vi "Get Software Set Config.vi"(8 "error in (no error)":errorcluster) -> (0 "error out":errorcluster, 2 "add on guids":string[](array[string]), 3 "software set guid":string)   [LabVIEW 2013]
uses:
  globals/Globals.vi
  <vilib>/Utility/config.llb/Read Key (String).vi
  <vilib>/Utility/sysdir.llb/Get System Directory.vi
  <vilib>/Utility/config.llb/NI_LVConfig.lvlib
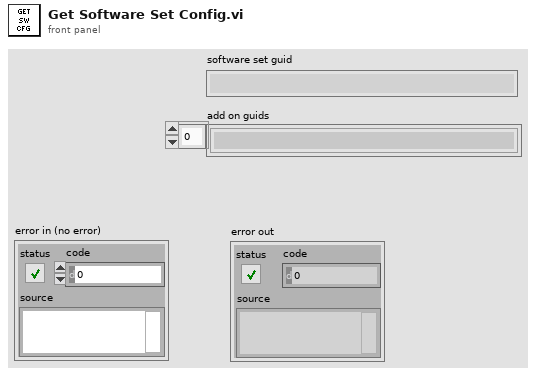
[diagram p1: front panel]
types:
  T1 = typedef "NI_LVConfig.lvlib/Config Data RefNum.ctl" = refnum<k1>
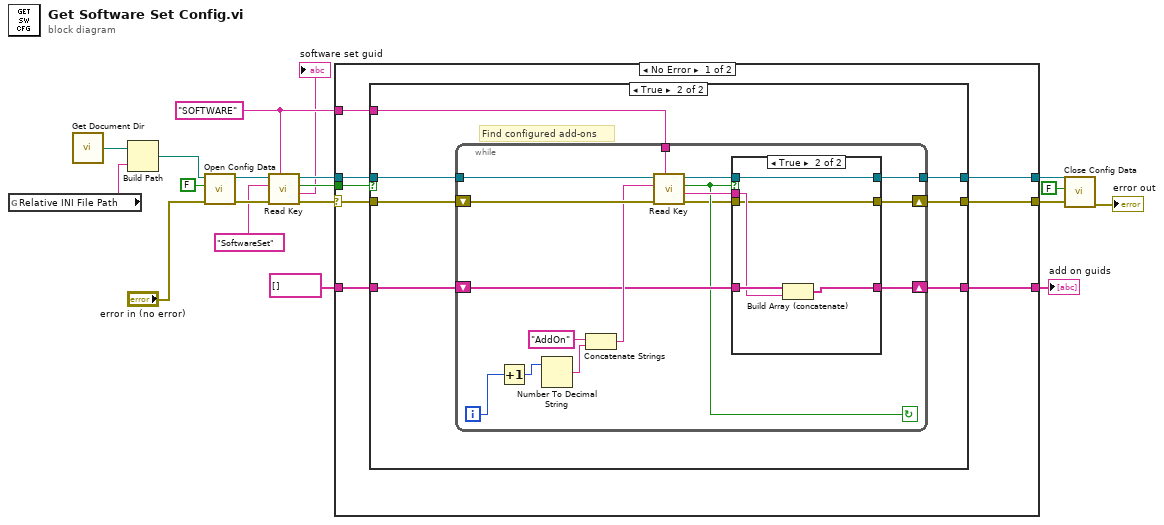
[diagram p0: block diagram]
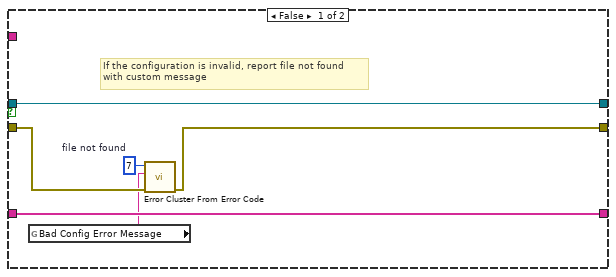
[diagram p2: hidden frame]
diagram:
  w19 = "SOFTWARE" ("section")
  n1 = global read "Globals.vi" "Relative INI File Path"() -> (w13:string)
  n2 = call "Get Document Dir.vi"() -> ("document dir"=w14:path)
  n3 = Build Path(base path=w14, name or relative path=w13) -> (appended path=w12:path)
  n4 = call <vilib>:"Open Config Data.vi"("error in (no error)"="error in (no error)", "create file if necessary (T)"=FALSE, "configuration file path"=w12) -> ("error out"=w16:errorcluster, "refnum"=w17:T1)  [unwired: 6 in, 1 out]
  n5 = call-poly <vilib>:"Read Key.vi"("section"=w19, "error in (no error)"=w16, "key"="SoftwareSet", "refnum"=w17) -> ("error out"=w9:errorcluster, "value"=→"software set guid":string, "found?"=w11:bool, "refnum out"=w10:T1)  [unwired: 4 in]
  n6 = case shown="No Error" w9 {
    selector: w9 -> [w25 w66]
    tunnel: w11 -> [w27 _]
    tunnel: w10 -> [w26 w67]
    tunnel: w19 -> [w24 _]
    tunnel: string[] [] -> [w23 w65]
    tunnel: [w22 w65] -> w5
    tunnel: [w21 w66] -> w4
    tunnel: [w20 w67] -> w3
    frame No Error {
      n7 = case shown="True" w27 {
        tunnel: w26 -> [w28 w40]
        tunnel: w25 -> [w31 w39]
        tunnel: w24 -> [_ w38]
        tunnel: w23 -> [w33 w37]
        tunnel: [w33 w36] -> w22
        tunnel: [w29 w35] -> w21
        tunnel: [w28 w34] -> w20
        frame False {
          w32 = 7  # file not found
          # "If the configuration is invalid, report file not found\nwith custom message"
          n8 = global read "Globals.vi" "Bad Config Error Message"() -> (w30:string)
          n9 = call <vilib>:"Error Cluster From Error Code.vi"("error in (no error)"=w31, "error message (\"\")"=w30, "error code (0)"=w32) -> ("error out"=w29:errorcluster)  [unwired: 6 in]
        }
        frame True {
          # "Find configured add-ons"
          n10 = while {
            tunnel: w40 -> [w50]
            shift-right: [w41] -> w35
            shift-left: w39 -> [w51]
            tunnel: w38 -> [w52]
            shift-right: [w45] -> w36
            shift-left: w37 -> [w48]
            tunnel: [w44] -> w34
            i -> [w56]
            stop <- w43 continue-if-true
            n11 = Increment(x=w56) -> (x+1=w55:i32)
            n12 = Number To Decimal String(number=w55) -> (decimal integer string=w53:string)  [unwired: 1 in]
            n13 = Concatenate Strings("AddOn" ("key"), w53) -> (w49:string)
            n14 = call-poly <vilib>:"Read Key.vi"("section"=w52, "error in (no error)"=w51, "key"=w49, "refnum"=w50) -> ("error out"=w42:errorcluster, "value"=w46:string, "found?"=w43:bool, "refnum out"=w47:T1)  [unwired: 4 in]
            n15 = case shown="True" w43 {
              tunnel: w48 -> [w58 w63]
              tunnel: [w59 w64] -> w44
              tunnel: w47 -> [w59 w64]
              tunnel: w46 -> [_ w62]
              tunnel: [w58 w61] -> w45
              tunnel: w42 -> [w57 w60]
              tunnel: [w57 w60] -> w41
              frame False {
              }
              frame True {
                n16 = Build Array (concatenate)(w63, w62) -> (w61:string[])
              }
            }
          }
        }
      }
    }
    frame Error {
    }
  }
  "add on guids" <- w5
  n17 = call <vilib>:"Close Config Data.vi"("error in (no error)"=w4, "write file if changed (T)"=FALSE, "refnum"=w3) -> ("error out"=→"error out":errorcluster)  [unwired: 7 in, 1 out]
